vi "solar_misc CPU Memory.vi"(8 "error in (no error)":errorcluster, 9 "Close Refnums? (F)":bool) -> (0 "error out":errorcluster, 1 "Free (MB)":dbl format="%#f", 2 "Available (MB)":dbl format="%#f", 3 "Memory Usage (%)":dbl, 4 "Committed (MB)":dbl format="%#f")   [LabVIEW 2018]
doc: "This returns the memory utilization in percent used of the total RAM, available, free and committed (i.e. used) using the .NET System.Diagnostics.PerformanceCounter API."
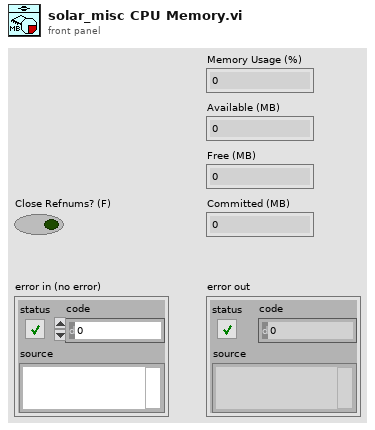
[diagram p1: front panel]
types:
  T1 = cluster{"Category":string, "Counter":string, "Instance":string}[]
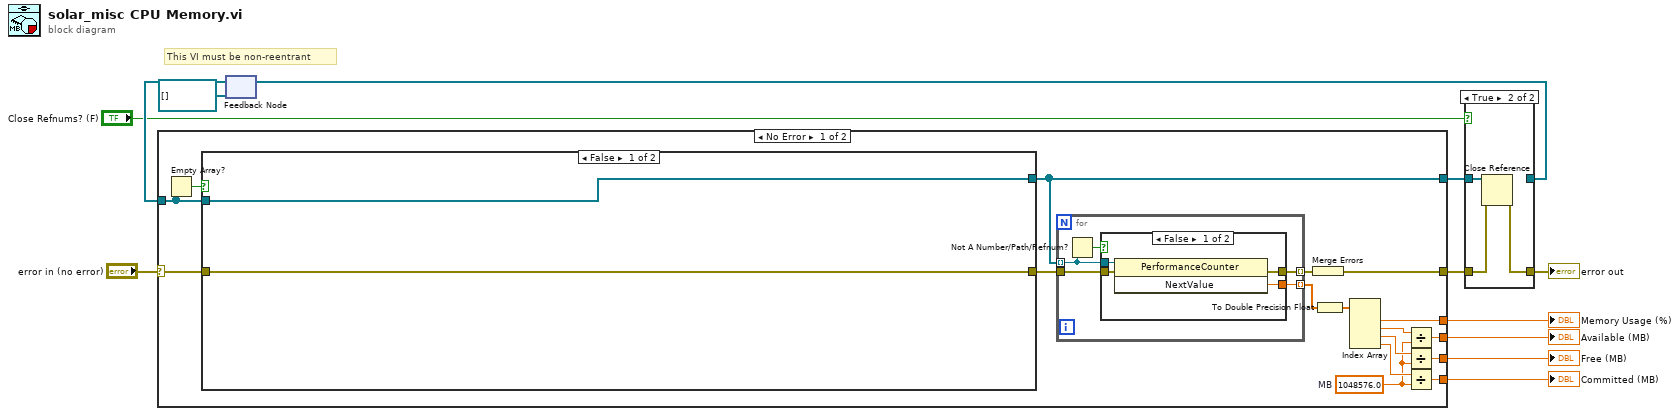
[diagram p0: block diagram]
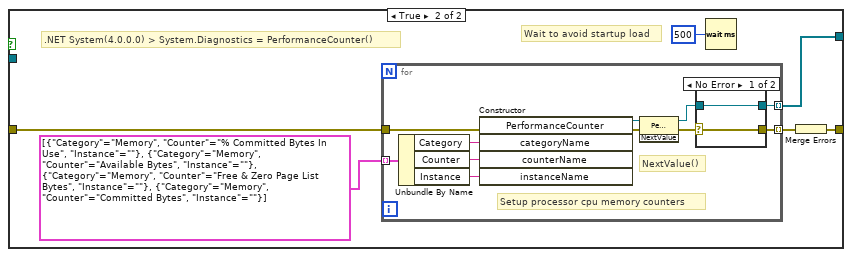
[diagram p3: hidden frame]
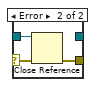
[diagram p4: hidden frame]
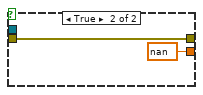
[diagram p5: hidden frame]
diagram:
  # "This VI must be non-reentrant"
  n1 = feedback #1(refnum<k24>[] []) -> (w12:refnum<k24>[])
  n2 = case shown="No Error" "error in (no error)" {
    selector: "error in (no error)" -> [w29 w66]
    tunnel: [w14 w65] -> w4
    tunnel: w12 -> [w28 w65]
    tunnel: [w13 w66] -> w3
    tunnel: [w22 _] -> w9
    tunnel: [w17 _] -> w8
    tunnel: [w16 _] -> w7
    tunnel: [w15 _] -> w6
    frame No Error {
      w18 = 1048576.0  # MB
      n3 = Empty Array?(array=w28) -> (empty?=w27:bool)
      n4 = case shown="False" w27 {
        tunnel: [w31 w32] -> w14
        tunnel: w28 -> [w31 _]
        tunnel: w29 -> [w30 w34]
        tunnel: [w30 w36] -> w26
        frame False {
        }
        frame True {
          # "Wait to avoid startup load"
          # ".NET System(4.0.0.0) > System.Diagnostics = PerformanceCounter()"
          n5 = for {
            tunnel: [w40] -> w37 mode=indexing
            tunnel: [w38] -> w32 mode=indexing
            tunnel: w34 -> [w46]
            tunnel: T1 [{"Category"="Memory", "Counter"="% Committed Bytes In Use", "Instance"=""}, {"Category"="Memory", "Counter"="Available Bytes", "Instance"=""}, {"Category"="Memory", "Counter"="Free & Zero Page List Bytes", "Instance"=""}, {"Category"="Memory", "Counter"="Committed Bytes", "Instance"=""}] ("Monitor") -> [w45] mode=indexing
            # "Setup processor cpu memory counters"
            # "NextValue()"
            n6 = Unbundle By Name(w45) -> ("Category"=w44:string, "Counter"=w43:string, "Instance"=w42:string)
            n7 = constructor class="PerformanceCounter"(error in=w46, "categoryName"=w44, "counterName"=w43, "instanceName"=w42) -> (reference out=w47:refnum<k24>, error out=w48:errorcluster)  [unwired: 2 in, 4 out]
            n8 = invoke class="PerformanceCounter" method="NextValue"(reference=w47, error in=w48) -> (reference out=w39:refnum<k24>, error out=w41:errorcluster)  [unwired: 1 in, 1 out]
            n9 = case shown="No Error" w41 {
              selector: w41 -> [w50 w53]
              tunnel: [w50 w52] -> w40
              tunnel: w39 -> [w49 w51]
              tunnel: [w49 _] -> w38
              frame No Error {
              }
              frame Error {
                n10 = Close Reference(reference=w51, error in (no error)=w53) -> (error out=w52:errorcluster)
              }
            }
          }
          n11 = Wait (ms)(milliseconds to wait=u32 500) -> ()  [unwired: 1 out]
          n12 = Merge Errors(w37) -> (w36:errorcluster)
        }
      }
      n13 = for {
        tunnel: w14 -> [w55] mode=indexing
        tunnel: w26 -> [w58]
        tunnel: [w57] -> w24 mode=indexing
        tunnel: [w56] -> w25 mode=indexing
        n14 = Not A Number/Path/Refnum?(number/path/refnum=w55) -> (NaN/Path/Refnum?=w54:bool)
        n15 = case shown="False" w54 {
          tunnel: w55 -> [w62 _]
          tunnel: w58 -> [w61 w64]
          tunnel: [w60 sgl nan ("NextValue")] -> w57
          tunnel: [w59 w64] -> w56
          frame False {
            n16 = invoke class="PerformanceCounter" method="NextValue"(reference=w62, error in=w61) -> (error out=w59:errorcluster, "NextValue"=w60:sgl)  [unwired: 1 in, 1 out]
          }
          frame True {
          }
        }
      }
      n17 = Merge Errors(w25) -> (w13:errorcluster)
      n18 = To Double Precision Float(number=w24) -> (double precision float=w23:dbl[])
      n19 = Index Array(array=w23) -> (element #1=w22:dbl, element #2=w21:dbl, element #3=w20:dbl, element #4=w19:dbl)  [unwired: 4 in]
      n20 = Divide(x=w21, y=w18) -> (x/y=w17:dbl)
      n21 = Divide(x=w20, y=w18) -> (x/y=w16:dbl)
      n22 = Divide(x=w19, y=w18) -> (x/y=w15:dbl)
    }
    frame Error {
    }
  }
  "Memory Usage (%)" <- w9
  "Free (MB)" <- w7
  "Available (MB)" <- w8
  "Committed (MB)" <- w6
  n23 = case shown="True" "Close Refnums? (F)" {
    tunnel: w4 -> [w68 w71]
    tunnel: [w68 _] -> w1
    tunnel: [w67 w69] -> w2
    tunnel: w3 -> [w67 w70]
    frame False {
    }
    frame True {
      n24 = Close Reference(reference=w71, error in (no error)=w70) -> (error out=w69:errorcluster)
    }
  }
  "error out" <- w2
  n25 = feedback-in #1(w1) -> ()
